vi "Atoms to GULP File.vi"(6 "Potentials":T2={"Potential Used"="sw2", "Potential Details"=[{"Atom 1"="Cd core", "Atom 2"="Te core", "Parameters"=[7.261088, 2.51, 23.9020768], "Range Min (A)"=0.0, "Range Max (A)"=4.518}, {"Atom 1"="Cd core", "Atom 2"="Cd core", "Parameters"=[5.327778, 2.51, 34.9560927], "Range Min (A)"=0.0, "Range Max (A)"=4.518}, {"Atom 1"="Te core", "Atom 2"="Te core", "Parameters"=[8.385745, 2.51, 26.4780396], "Range Min (A)"=0.0, "Range Max (A)"=4.518}]}, 8 "Lattice Vectors":T1={"Lattice Vector Type"=enum."Vectors", "DoF to Allow Relaxation?"=[1, 1, 1, 1, 1, 1]}, 9 "Title and Comments":string, 10 "Relaxation Type":string(combo)="conv opti", 11 "Structure":T3={"Structure Name"="CdTe", "Lattice vector a"=[6.615785553057252, 0.0, 0.0], "Lattice vector b"=[0.0, 6.615785553057252, 0.0], "Lattice vector c"=[0.0, 0.0, 6.615785553057252], "Atoms Array"=[{"Atom Name"="Cd", "Positions (Direct)"=[[0.0, 0.0, 0.0], [0.0, 0.5, 0.5], [0.5, 0.0, 0.5], [0.5, 0.5, 0.0]], "Positions (Cartesian)"=[[0.0, 0.0, 0.0], [0.0, 3.307892776528626, 3.307892776528626], [3.307892776528626, 0.0, 3.307892776528626], [3.307892776528626, 3.307892776528626, 0.0]]}, {"Atom Name"="Te", "Positions (Direct)"=[[0.25, 0.25, 0.25], [0.75, 0.75, 0.25], [0.75, 0.25, 0.75], [0.25, 0.75, 0.75]], "Positions (Cartesian)"=[[1.653946388264313, 1.653946388264313, 1.653946388264313], [4.96183916479294, 4.96183916479294, 1.653946388264313], [4.96183916479294, 1.653946388264313, 4.96183916479294], [1.653946388264313, 4.96183916479294, 4.96183916479294]]}], "# of atoms"=8}) -> (3 "GULP File":string)   [LabVIEW 2010]
uses:
  <vilib>/Utility/error.llb/whitespace.ctl
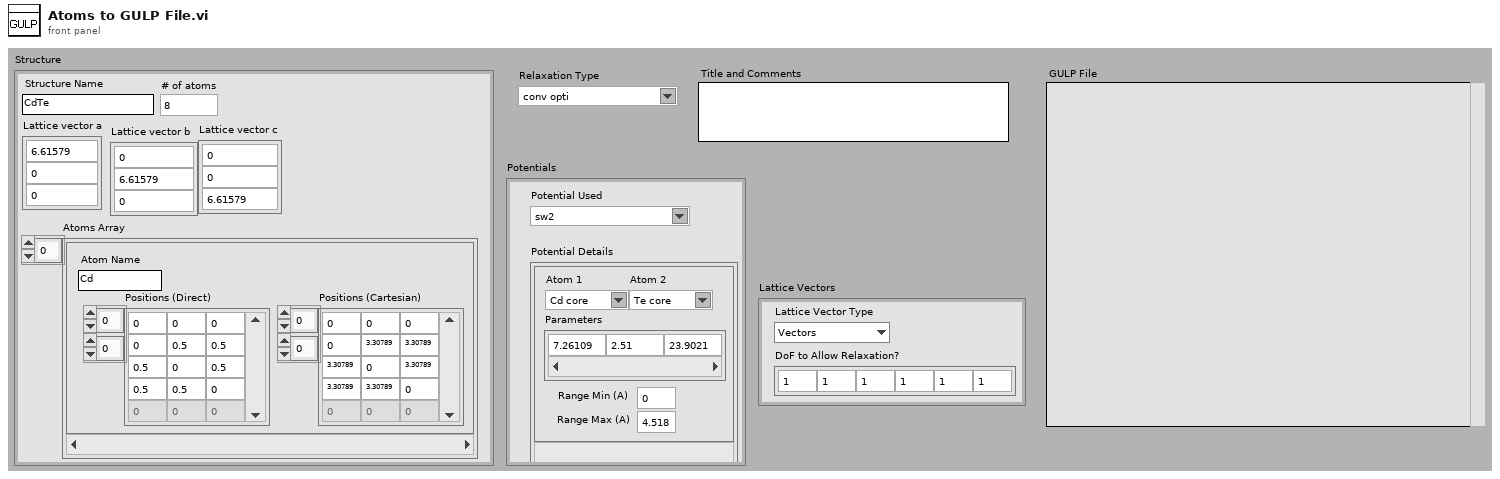
[diagram p1: front panel]
types:
  T1 = cluster{"Lattice Vector Type":enum16{"Vectors", "Cell"}, "DoF to Allow Relaxation?":i32[]}
  T2 = cluster{"Potential Used":string, "Potential Details":cluster{"Atom 1":string, "Atom 2":string, "Parameters":dbl[], "Range Min (A)":dbl, "Range Max (A)":dbl}[]}
  T3 = cluster{"Structure Name":string, "Lattice vector a":dbl[], "Lattice vector b":dbl[], "Lattice vector c":dbl[], "Atoms Array":cluster{"Atom Name":string, "Positions (Direct)":dbl[][], "Positions (Cartesian)":dbl[][]}[], "# of atoms":i32}
  T4 = typedef "whitespace.ctl" = u16
  T5 = cluster{"Atom Name":string, "Positions (Direct)":dbl[][], "Positions (Cartesian)":dbl[][]}[]
  T6 = cluster{"Atom 1":string, "Atom 2":string, "Parameters":dbl[], "Range Min (A)":dbl, "Range Max (A)":dbl}[]
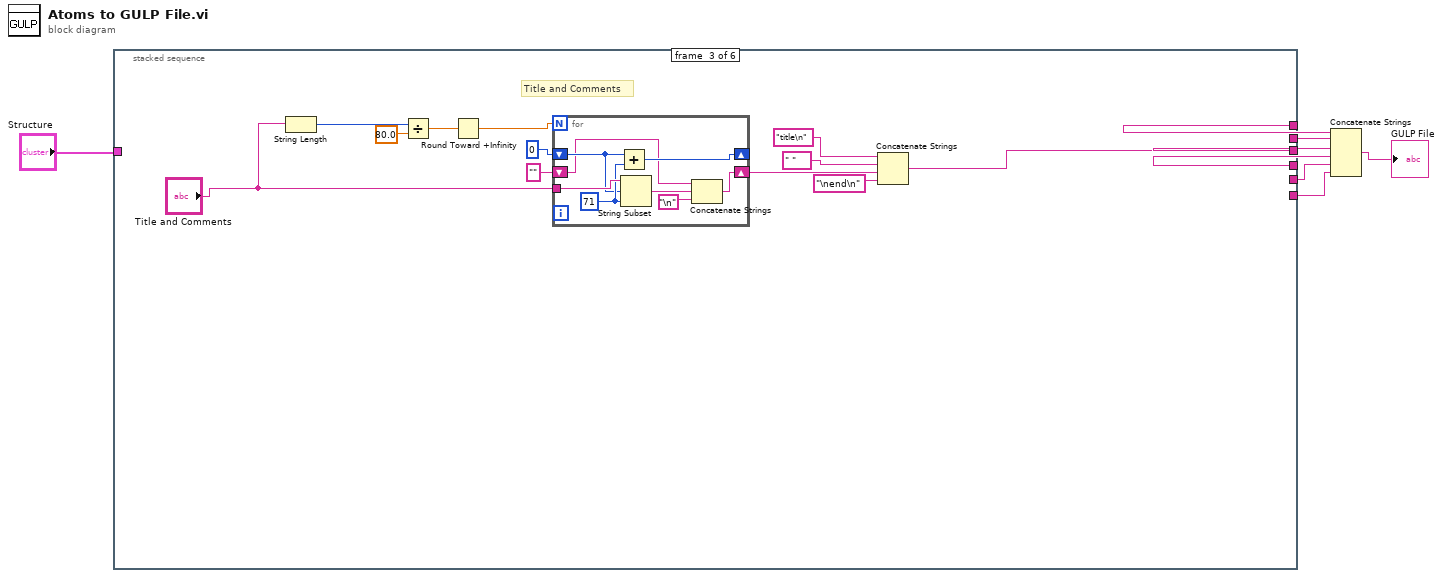
[diagram p0: block diagram]
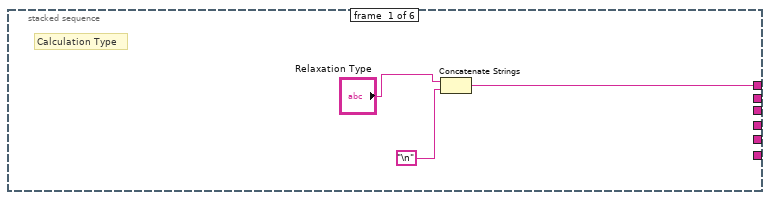
[diagram p2: hidden frame]
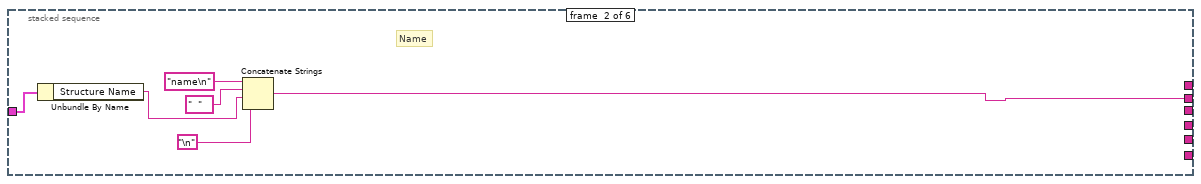
[diagram p3: hidden frame]
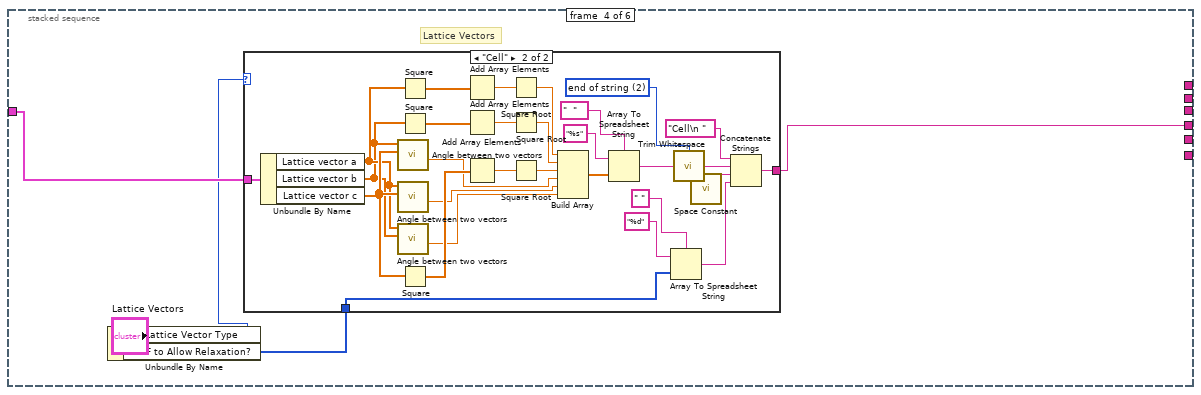
[diagram p4: hidden frame]
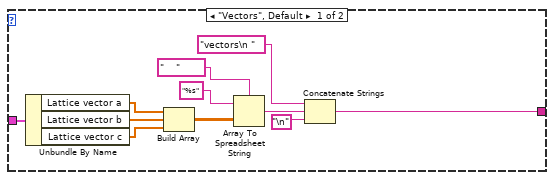
[diagram p5: hidden frame]
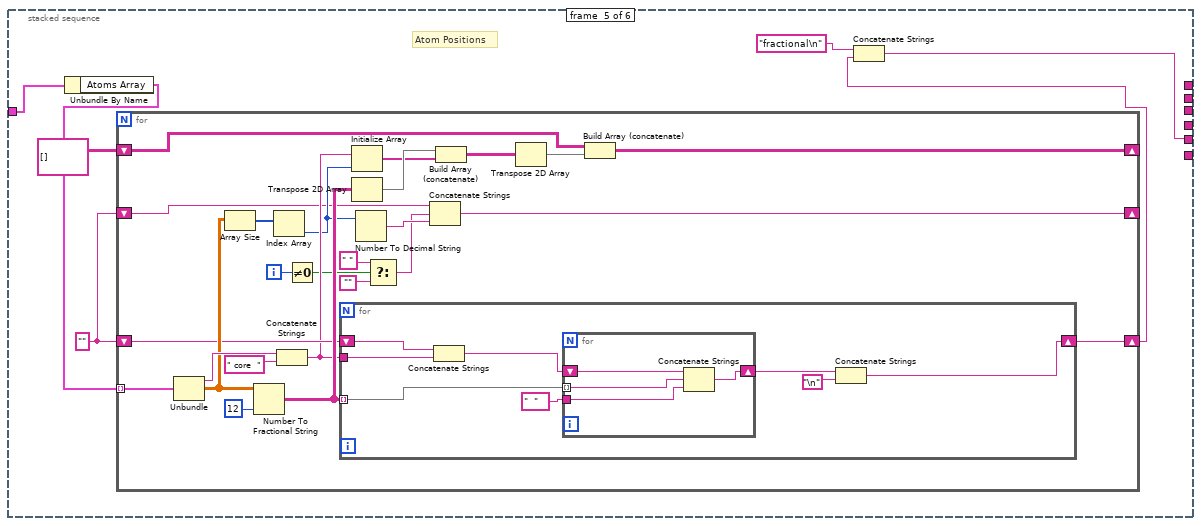
[diagram p6: hidden frame]
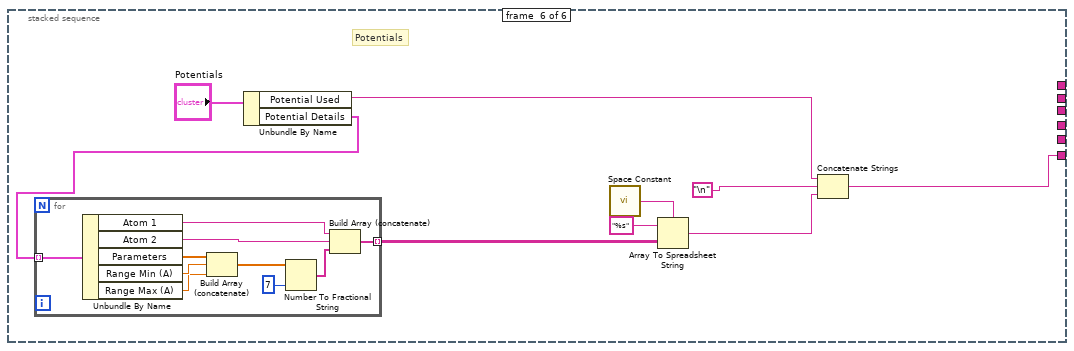
[diagram p7: hidden frame]
diagram:
  n1 = stacked-sequence {
    tunnel: [w9 _ _ _ _ _] -> w7
    tunnel: "Structure" -> [_ w17 _ w42 w86 _]
    tunnel: [_ w12 _ _ _ _] -> w6
    tunnel: [_ _ w19 _ _ _] -> w5
    tunnel: [_ _ _ w41 _ _] -> w4
    tunnel: [_ _ _ _ w83 _] -> w3
    tunnel: [_ _ _ _ _ w130] -> w2
    frame #0 {
      # "Calculation Type"
      n2 = Concatenate Strings("Relaxation Type", "\n") -> (w9:string)
    }
    frame #1 {
      # "Name"
      n3 = Unbundle By Name(w17) -> ("Structure Name"=w14:string)
      n4 = Concatenate Strings("name\n" ("string"), "  ", w14, "\n") -> (w12:string)
    }
    frame #2 {
      # "Title and Comments"
      n5 = String Length(string="Title and Comments") -> (length=w24:i32)
      n6 = Divide(x=w24, y=80.0) -> (x/y=w25:dbl)
      n7 = Round Toward +Infinity(x=w25) -> (ceil(x): smallest int >= x=w26:dbl)
      n8 = for {
        N: w26 -> [_]
        tunnel: "Title and Comments" -> [w37]
        shift-right: [w35] -> _
        shift-left: 0 -> [w34]
        shift-right: [w31] -> w29
        shift-left: "" -> [w30]
        w36 = 71 ("length (rest)")
        n9 = Add(x=w34, y=w36) -> (x+y=w35:i32)
        n10 = String Subset(string=w37, offset (0)=w34, length (rest)=w36) -> (substring=w33:string)
        n11 = Concatenate Strings(w30, w33, "\n") -> (w31:string)
      }
      n12 = Concatenate Strings("title\n" ("string"), " ", w29, "\nend\n" ("string")) -> (w19:string)
    }
    frame #3 {
      # "Lattice Vectors"
      n13 = Unbundle By Name("Lattice Vectors") -> ("Lattice Vector Type"=w39:enum16{"Vectors", "Cell"}, "DoF to Allow Relaxation?"=w38:i32[])
      n14 = case shown="\"Cell\"" w39 {
        tunnel: w42 -> [w53 w73]
        tunnel: [w43 w62] -> w41
        tunnel: w38 -> [_ w54]
        frame "Vectors", Default {
          n15 = Unbundle By Name(w53) -> ("Lattice vector a"=w50:dbl[], "Lattice vector b"=w49:dbl[], "Lattice vector c"=w48:dbl[])
          n16 = Build Array(w50, w49, w48) -> (w47:dbl[][])
          n17 = Array To Spreadsheet String(delimiter (Tab)="    " ("string"), array=w47, 3:"%s" ("format string")) -> (spreadsheet string=w45:string)
          n18 = Concatenate Strings("vectors\n " ("string"), w45, "\n") -> (w43:string)
        }
        frame "Cell" {
          w57 = T4 2 items=["both", "start of string", "end of string"] ("location (both)")
          n19 = Unbundle By Name(w73) -> ("Lattice vector a"=w69:dbl[], "Lattice vector b"=w68:dbl[], "Lattice vector c"=w71:dbl[])
          n20 = call "Angle between two vectors.vi"("Vector 2"=w71, "Vector 1"=w68) -> ("Angle (Degrees)"=w72:dbl)  [unwired: 7 in, 2 out]
          n21 = call "Angle between two vectors.vi"("Vector 2"=w71, "Vector 1"=w69) -> ("Angle (Degrees)"=w70:dbl)  [unwired: 7 in, 2 out]
          n22 = call "Angle between two vectors.vi"("Vector 2"=w68, "Vector 1"=w69) -> ("Angle (Degrees)"=w67:dbl)  [unwired: 7 in, 2 out]
          n23 = Square(x=w69) -> (x^2=w82:dbl[])
          n24 = Square(x=w68) -> (x^2=w79:dbl[])
          n25 = Square(x=w71) -> (x^2=w78:dbl[])
          n26 = Add Array Elements(numeric array=w82) -> (sum=w81:dbl)
          n27 = Add Array Elements(numeric array=w79) -> (sum=w80:dbl)
          n28 = Add Array Elements(numeric array=w78) -> (sum=w77:dbl)
          n29 = Square Root(x=w81) -> (sqrt(x)=w76:dbl)
          n30 = Square Root(x=w80) -> (sqrt(x)=w75:dbl)
          n31 = Square Root(x=w77) -> (sqrt(x)=w74:dbl)
          n32 = Build Array(w76, w75, w74, w72, w70, w67) -> (w64:dbl[])
          n33 = Array To Spreadsheet String(delimiter (Tab)="  " ("string"), array=w64, 3:"%s" ("format string")) -> (spreadsheet string=w58:string)
          n34 = Array To Spreadsheet String(delimiter (Tab)=" ", array=w54, 3:"%d" ("format string")) -> (spreadsheet string=w59:string)
          n35 = call <vilib>:"Trim Whitespace.vi"("string"=w58, "location (both)"=w57) -> ("trimmed string"=w56:string)
          n36 = call <vilib>:"Space Constant.vi"() -> ("String"=w55:string)
          n37 = Concatenate Strings("Cell\n " ("string"), w56, w55, w59) -> (w62:string)
        }
      }
    }
    frame #4 {
      w88 = ""
      # "Atom Positions"
      n38 = Unbundle By Name(w86) -> ("Atoms Array"=w85:T5)
      n39 = for {
        tunnel: w85 -> [w114] mode=indexing
        shift-right: [w111] -> _
        shift-left: string[][] [] -> [w110]
        shift-right: [w103] -> w84
        shift-left: w88 -> [w102]
        shift-right: [w94] -> _
        shift-left: w88 -> [w93]
        i -> [w97]
        n40 = Unbundle(w114) -> ("Atom Name"=w113:string, "Positions (Direct)"=w105:dbl[][])  [unwired: 1 out]
        n41 = Array Size(array=w105) -> (size(s)=w112:i32[])
        n42 = Number To Fractional String(number=w105, precision (6)=i16 12) -> (F-format string=w104:string[][])  [unwired: 2 in]
        n43 = Index Array(array=w112) -> (element=w100:i32)  [unwired: 1 in]
        n44 = Concatenate Strings(w113, " core  " ("string")) -> (w101:string)
        n45 = Not Equal To 0?(x=w97) -> (x != 0?=w99:bool)
        n46 = for {
          tunnel: w104 -> [w122] mode=indexing
          shift-right: [w120] -> w103
          shift-left: w102 -> [w117]
          tunnel: w101 -> [w116]
          n47 = Concatenate Strings(w117, w116) -> (w115:string)
          n48 = for {
            tunnel: w122 -> [w125] mode=indexing
            shift-right: [w124] -> w118
            shift-left: w115 -> [w123]
            tunnel: "  " ("delimiter (Tab)") -> [w126]
            n49 = Concatenate Strings(w123, w125, w126) -> (w124:string)
          }
          n50 = Concatenate Strings(w118, "\n") -> (w120:string)
        }
        n51 = Initialize Array(w101, w100) -> (w108:string[])
        n52 = Transpose 2D Array(2D array=w104) -> (transposed array=w109:string[][])
        n53 = Number To Decimal String(number=w100) -> (decimal integer string=w96:string)  [unwired: 1 in]
        n54 = Select(t=" " ("string"), s=w99, f="") -> (s? t:f=w95:string)
        n55 = Concatenate Strings(w93, w95, w96) -> (w94:string)
        n56 = Build Array (concatenate)(w109, w108) -> (w107:string[][])
        n57 = Transpose 2D Array(2D array=w107) -> (transposed array=w106:string[][])
        n58 = Build Array (concatenate)(w110, w106) -> (w111:string[][])
      }
      n59 = Concatenate Strings("fractional\n" ("string"), w84) -> (w83:string)
    }
    frame #5 {
      # "Potentials"
      n60 = Unbundle By Name("Potentials") -> ("Potential Used"=w128:string, "Potential Details"=w127:T6)
      n61 = for {
        tunnel: w127 -> [w145] mode=indexing
        tunnel: [w136] -> w134 mode=indexing
        n62 = Unbundle By Name(w145) -> ("Atom 1"=w143:string, "Atom 2"=w142:string, "Parameters"=w140:dbl[], "Range Min (A)"=w139:dbl, "Range Max (A)"=w138:dbl)
        n63 = Build Array (concatenate)(w140, w139, w138) -> (w137:dbl[])
        n64 = Number To Fractional String(number=w137, precision (6)=i16 7) -> (F-format string=w141:string[])  [unwired: 2 in]
        n65 = Build Array (concatenate)(w143, w142, w141) -> (w136:string[])
      }
      n66 = call <vilib>:"Space Constant.vi"() -> ("String"=w133:string)
      n67 = Array To Spreadsheet String(delimiter (Tab)=w133, array=w134, 3:"%s" ("format string")) -> (spreadsheet string=w131:string)
      n68 = Concatenate Strings(w128, "\n", w131) -> (w130:string)
    }
  }
  n69 = Concatenate Strings(w7, w6, w5, w4, w3, w2) -> (→"GULP File":string)
